vi "Reverse Byte Order (SubVI).vi"(11 "Data In":u64) -> (3 "Data Out":u64)   [LabVIEW 2015]
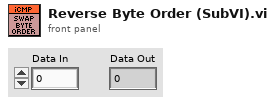
[diagram p1: front panel]
types:
  T1 = cluster{"Numeric Control":u8, "Numeric Control":u8, "Numeric Control":u8, "Numeric Control":u8, "Numeric Control":u8, "Numeric Control":u8, "Numeric Control":u8, "Numeric Control":u8}
  T2 = cluster{"[0]":u8, "[1]":u8, "[2]":u8, "[3]":u8, "[4]":u8, "[5]":u8, "[6]":u8, "[7]":u8}
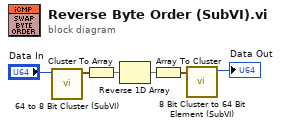
[diagram p0: block diagram]
diagram:
  n1 = call "64 to 8 Bit Cluster (SubVI).vi"("Data In"="Data In") -> ("Data Out"=w1:T1)  [unwired: 10 in]
  n2 = Cluster To Array(cluster=w1) -> (array=w2:u8[])
  n3 = Reverse 1D Array(array=w2) -> (reversed array=w4:u8[])
  n4 = Array To Cluster(array=w4) -> (cluster=w3:T2)
  n5 = call "8 Bit Cluster to 64 Bit Element (SubVI).vi"("Pixel Cluster"=w3) -> ("Pixel Data (64-Bit)"=→"Data Out":u64)  [unwired: 10 in]
